vi "Analog Input - N Channels - Continuous Sampling.vi"() -> ()   [LabVIEW 2019]
uses:
  <vilib>/myRIO/Common/Instrument Driver Framework/myRIO v1.0/UART/vis/myRIO v1.0 Close UART.vi
  <vilib>/myRIO/Instrument Drivers/Onboard IO/AI Continuous/vis/AI Continuous Smart Read.vi
  <vilib>/myRIO/Common/Instrument Driver Framework/Utilities/vis/FPGA Ref Manager.vi
  <vilib>/myRIO/Common/Instrument Driver Framework/ELVIS III v1.0/ELVIS III v1.0 Reset FPGA.vi
  <vilib>/myRIO/Common/Instrument Driver Framework/myRIO v1.0/IRQ/vis/myRIO v1.0 IRQ Info FGV.vi
  <vilib>/myRIO/Common/Instrument Driver Framework/myRIO v1.0/IRQ/vis/myRIO v1.0 Timer IRQ Info FGV.vi
  <vilib>/myRIO/Common/Instrument Driver Framework/myRIO v1.0/IRQ/vis/myRIO v1.0 ISR Agent.vi
  <vilib>/myRIO/Instrument Drivers/Utilities/vis/Reset Index.vi
  <vilib>/myRIO/Common/Instrument Driver Framework/myRIO v1.0/Resource Manager/vis/myRIO v1.0 Block Write Resource Manager.vi
  <vilib>/myRIO/Express VI/Onboard IO/AI/AI Express VI.xnode
  <vilib>/myRIO/Instrument Drivers/Utilities/Utilities.lvlib
  <vilib>/myRIO/Instrument Drivers/Onboard IO/AI Continuous/AI Continuous.lvlib
panel:
  in  "Stop":bool
  in  "Acquire Data":bool
  out "Analog Data":dbl[][](graph)
  # "ELVIS III Control IO"
  # "模拟输入N通道连续采集"
  # "Overview: Acquires voltage values continuously from Bank A, Channel 0 (A/AI0 & A/AI1) until the acquisition is stopped.\nInstructions:\n1. Connect A/AI0 & A/AI1 to a valid signal.\n2. Run the VI."
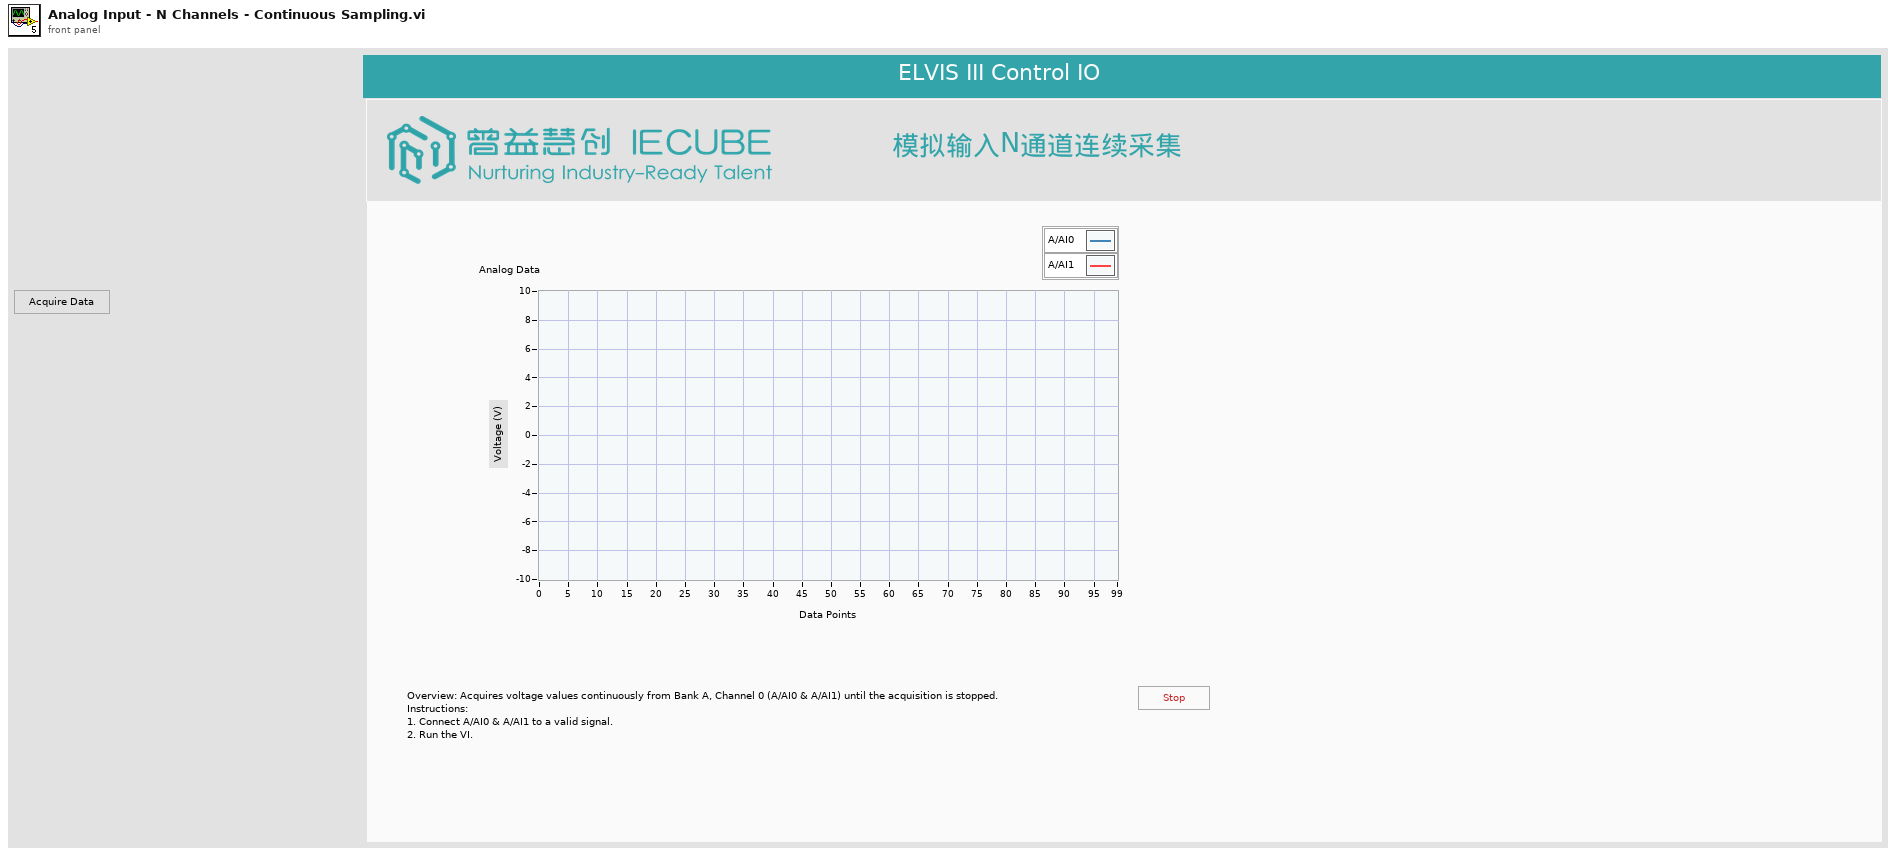
[diagram p1: front panel]
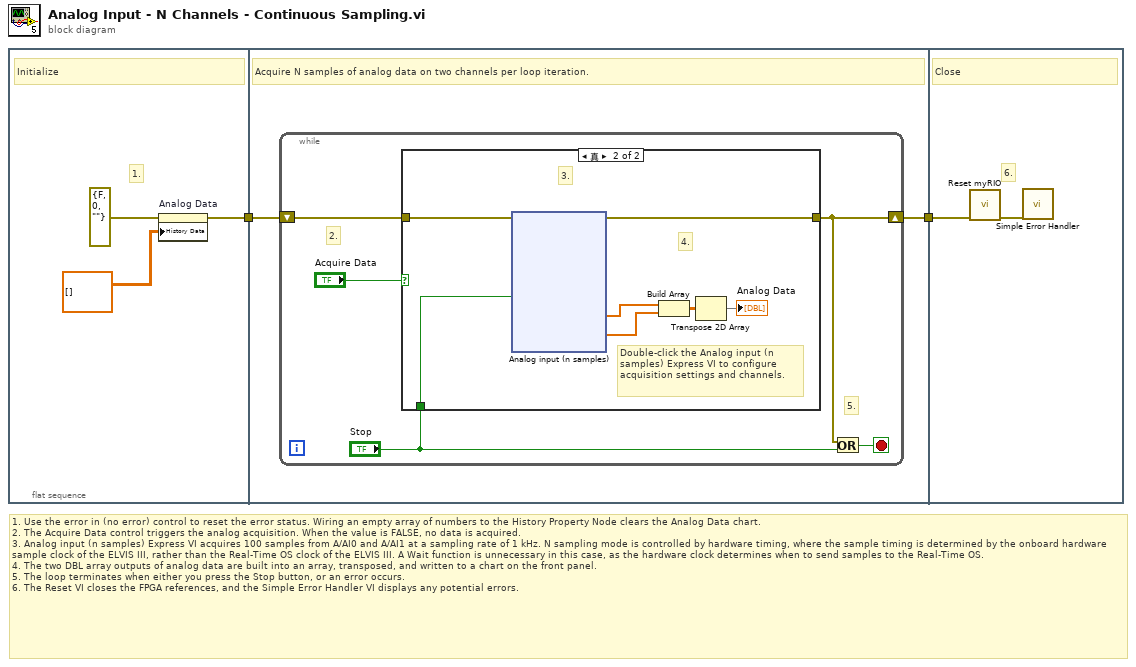
[diagram p0: block diagram]
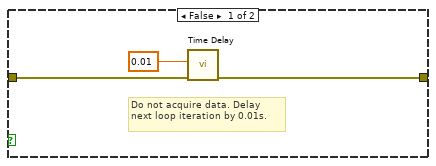
[diagram p2: hidden frame]
diagram:
  # "1. Use the error in (no error) control to reset the error status. Wiring an empty array of numbers to the History Property Node clears the Analog Data chart. \n2. The Acquire Data control triggers the analog acquisition. When the value is FALSE, no data is acquired.\n3. Analog input (n samples) Express VI acquires 100 samples from A/AI0 and A/AI1 at a sampling rate of 1 kHz. N sampling mode is controlled by hardware timing, where the sample timing is determined by the onboard hardware sample clock of the ELVIS III, rather than the Real-Time OS clock of the ELVIS III. A Wait function is unnecessary in this case, as the hardware clock determines when to send samples to the Real-Time OS.\n4. The two DBL array outputs of analog data are built into an array, transposed, and written to a chart on the front panel.\n5. The loop terminates when either you press the Stop button, or an error occurs.\n6. The Reset VI closes the FPGA references, and the Simple Error Handler VI displays any potential errors."
  n1 = flat-sequence {
    tunnel: [w4] -> w2
    tunnel: [w7] -> w1
    tunnel: w2 -> [w6]
    tunnel: w1 -> [w36]
    frame #0 {
      # "1."
      # "Initialize"
      n2 = property on="Analog Data" class="WFChart (严格)"(error in=errorcluster {"status"=FALSE, "code"=0, "source"=""} ("error in (no error)"), "History Data"=dbl[][] []) -> (error out=w4:errorcluster)  [unwired: 1 in, 1 out]
    }
    frame #1 {
      # "Acquire N samples of analog data on two channels per loop iteration."
      n3 = while {
        shift-right: [w10] -> w7
        shift-left: w6 -> [w11]
        stop <- w12 stop-if-true
        # "5."
        # "2."
        n4 = case shown="真" "Acquire Data" {
          tunnel: w11 -> [w14 w22]
          tunnel: [w13 w21] -> w10
          tunnel: "Stop" -> [_ w16]
          frame False {
            # "Do not acquire data. Delay next loop iteration by 0.01s."
            n5 = call "Time Delay"("error in (no error)"=w14, "Delay Time (s)"=0.01) -> ("error out"=w13:errorcluster)  [unwired: 9 in]
          }
          frame True {
            # "4."
            # "3."
            # "Double-click the Analog input (n samples) Express VI to configure acquisition settings and channels."
            n6 = xnode "Analog input (n samples)"("Stop?"=w16, "error in (no error)"=w22) -> ("A/AI0 (Continuous)"=w18:dbl[], "A/AI1 (Continuous)"=w17:dbl[], "error out"=w21:errorcluster)
            n7 = Build Array(w18, w17) -> (w20:dbl[][])
            n8 = Transpose 2D Array(2D array=w20) -> (transposed array=→"Analog Data":dbl[][])
          }
        }
        n9 = Or(x=w10, y="Stop") -> (x .or. y?=w12:bool)
      }
    }
    frame #2 {
      # "6."
      # "Close"
      n10 = call <vilib>:"Reset myRIO.vi"("error in (no error)"=w36) -> ("error out"=w35:errorcluster)  [unwired: 10 in]
      n11 = call <vilib>:"Simple Error Handler.vi"("error in (no error)"=w35) -> ()  [unwired: 4 in, 5 out]
    }
  }
